vi "Emballage_BDD_chargement_IDArticle_GPAO_FLATPROP.vi"(0 "filenames":string[](array[string]), 1 "taille":i32, 2 "repertoireConfigs":path, 3 "Refnum Ch":refnum<vi>, 7 "entrée d'erreur (pas d'erreur)":errorcluster, 12 "progress":refnum<vi>) -> (10 "Code_Barre_Fixe":string, 14 "affiche_code_barre_client":string, 16 "codification":string, 17 "melange_des_lots_possible":string, 18 "Indice":string, 19 "id_article":string, 20 "clc_designation":string, 21 "affiche-no-client":string, 22 "Tableau en sortie":string[][](array[string]), 23 "Nb_valve_par_carton":string, 24 "tableau ajouté":string[](array[string]), 25 "suffixe":string, 26 "INDICE_REV":string, 27 "sortie d'erreur":errorcluster)   [LabVIEW 2020]
uses:
  Modules/FS/60_FS_Controles/60_FS_SetGet.ctl
panel:
  out "code_barre_fixe_fin":string
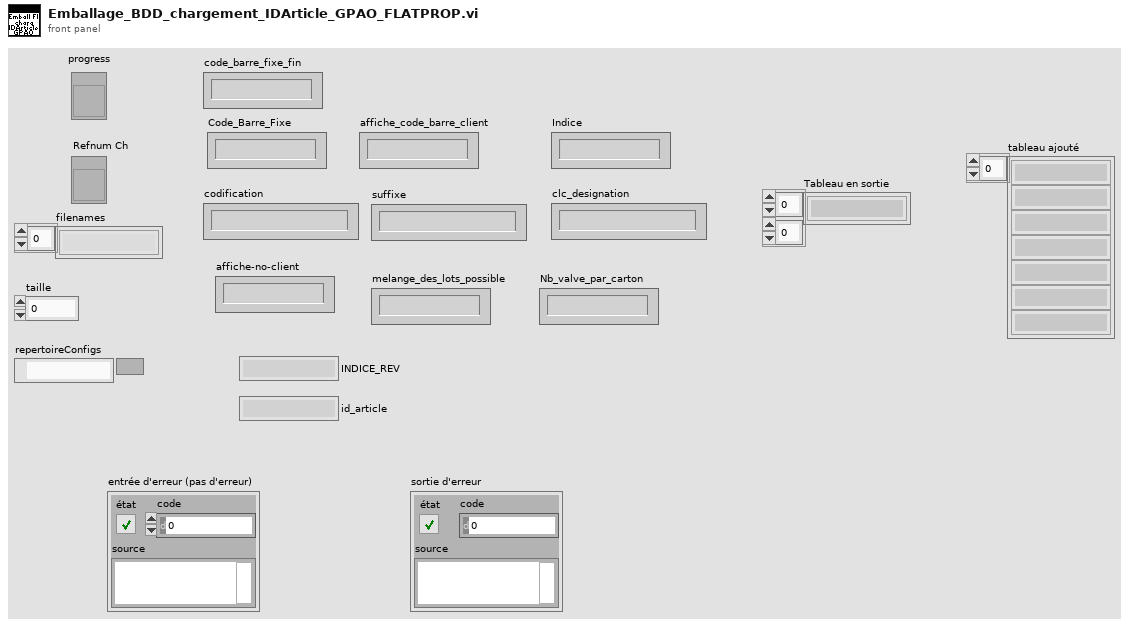
[diagram p1: front panel]
types:
  T1 = typedef "60_FS_SetGet.ctl" = enum16{"set", "get"}
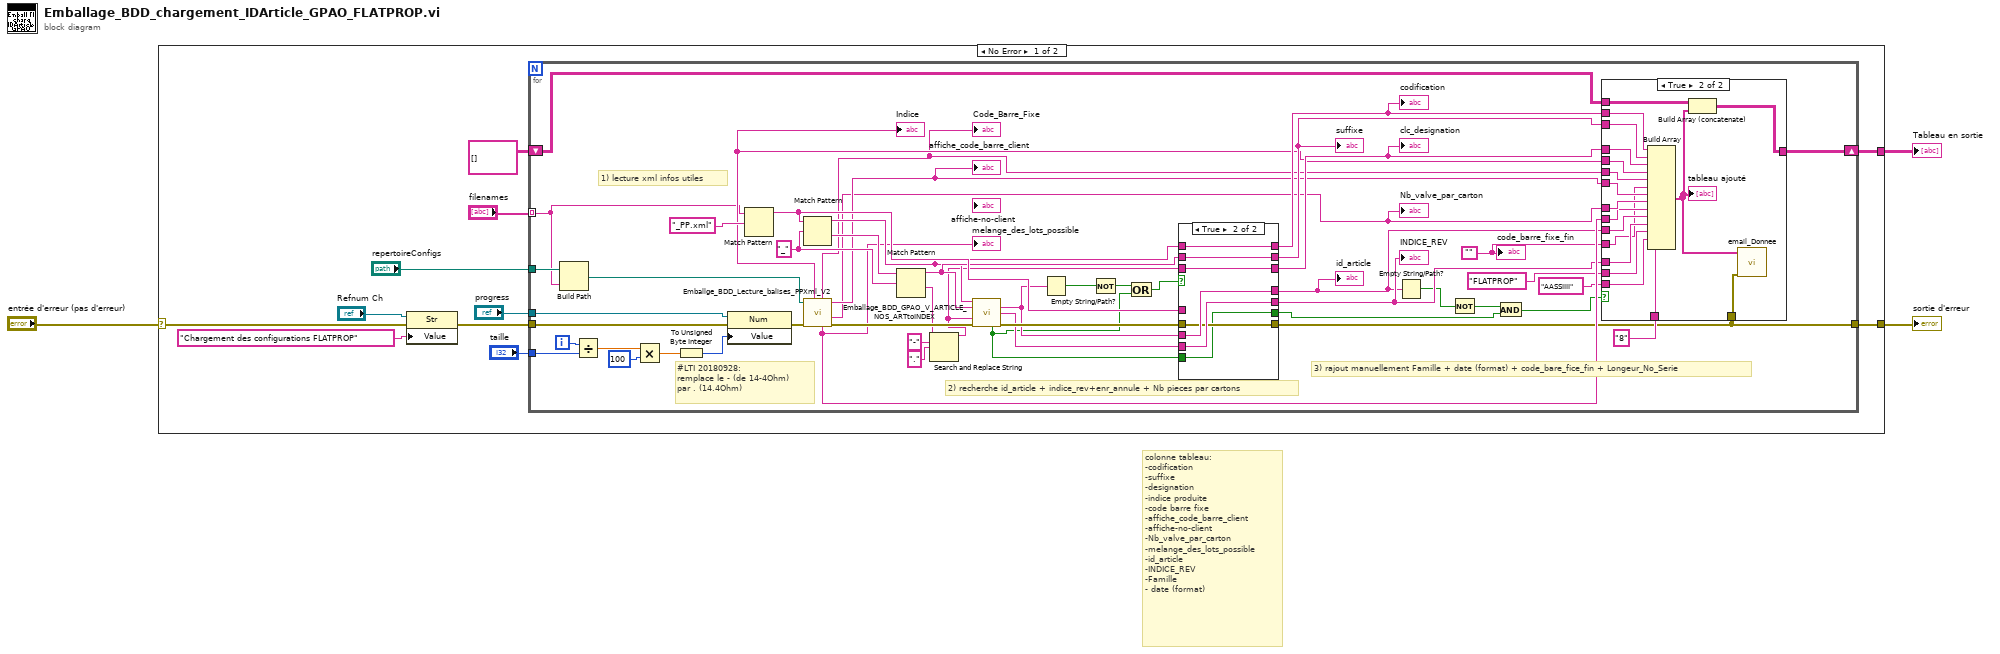
[diagram p0: block diagram]
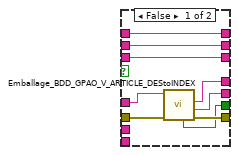
[diagram p3: hidden frame]
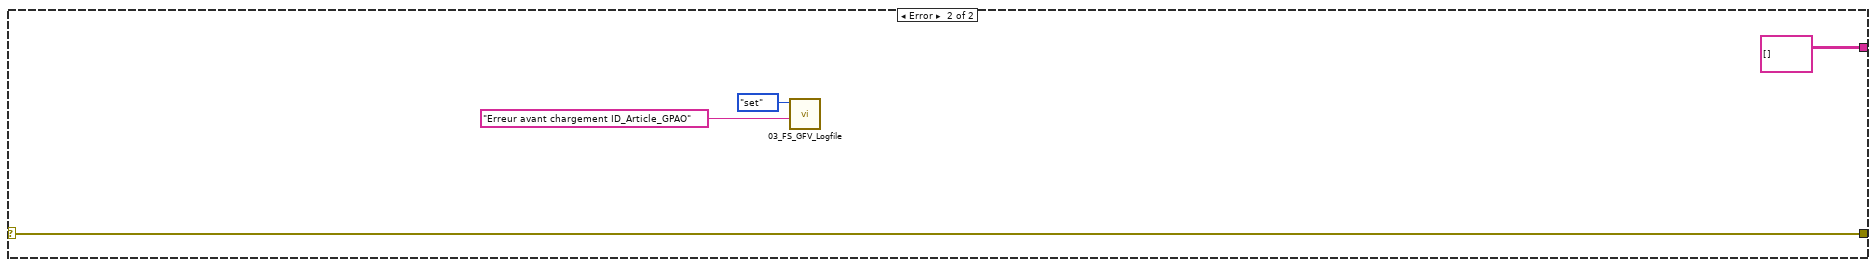
[diagram p4: hidden frame]
diagram:
  # "colonne tableau:\n-codification\n-suffixe\n-designation\n-indice produite\n-code barre fixe\n-affiche_code_barre_client\n-affiche-no-client\n-Nb_valve_par_carton\n-melange_des_lots_possible\n-id_article\n-INDICE_REV\n-Famille\n- date (format)"
  n1 = case shown="No Error" "entrée d'erreur (pas d'erreur)" {
    selector: "entrée d'erreur (pas d'erreur)" -> [w6 w104]
    tunnel: [w14 string[][] [] ("Tableau en entrée")] -> w3
    tunnel: [w9 w104] -> w1
    frame No Error {
      n2 = property class="Str"(reference="Refnum Ch", error in=w6, "Value"="Chargement des configurations FLATPROP" ("Valeur")) -> (error out=w5:errorcluster)  [unwired: 1 out]
      n3 = for {
        tunnel: "repertoireConfigs" -> [w65]
        tunnel: "filenames" -> [w19] mode=indexing
        tunnel: w5 -> [w35]
        tunnel: "taille" -> [w59]
        shift-right: [w38] -> w14
        shift-left: string[][] [] ("Tableau en entrée") -> [w39]
        tunnel: [w15] -> w9
        tunnel: "progress" -> [w33]
        i -> [w60]
        w23 = ""
        w51 = "_" ("expression régulière")
        # "#LTI 20180928:\nremplace le - (de 14-4Ohm)\npar . (14.4Ohm)"
        # "3) rajout manuellement Famille + date (format) + code_bare_fice_fin + Longeur_No_Serie"
        # "2) recherche id_article + indice_rev+enr_annule + Nb pieces par cartons"
        # "1) lecture xml infos utiles"
        n4 = Build Path(base path=w65, name or relative path=w19) -> (appended path=w64:path)
        n5 = Divide(x=w60, y=w59) -> (x/y=w61:dbl)
        n6 = Multiply(x=w61, y=u8 100) -> (x*y=w63:dbl)
        n7 = To Unsigned Byte Integer(number=w63) -> (unsigned 8bit integer=w36:u8)
        n8 = property class="Num"(reference=w33, error in=w35, "Value"=w36) -> (error out=w34:errorcluster)  [unwired: 1 out]
        n9 = Match Pattern(string=w19, regular expression="_PP.xml" ("expression régulière")) -> (before substring=w57:string)  [unwired: 1 in, 3 out]
        n10 = Match Pattern(string=w57, regular expression=w51) -> (before substring=w53:string, after substring=w52:string)  [unwired: 1 in, 2 out]
        n11 = call "Emballge_BDD_Lecture_balises_PPXml_V2.vi"("entrée d'erreur (pas d'erreur)"=w34, "appended path"=w64) -> ("sortie d'erreur"=w48:errorcluster, "Nb_valve_par_carton"=w16:string, "affiche_code_barre_client"=w42:string, "melange_des_lots_possible"=w41:string, "Code_Barre_Fixe"=w43:string, "Indice"=w44:string)  [unwired: 4 in]
        "affiche_code_barre_client" <- w42
        "melange_des_lots_possible" <- w41
        "Nb_valve_par_carton" <- w16
        "Code_Barre_Fixe" <- w43
        "Indice" <- w44
        n12 = Match Pattern(string=w52, regular expression=w51) -> (before substring=w54:string, after substring=w18:string)  [unwired: 1 in, 2 out]
        n13 = Search and Replace String(input string=w18, search string="-" ("chaîne recherchée"), replace string="." ("chaîne de remplacement (\"\")")) -> (result string=w17:string)  [unwired: 5 in, 3 out]
        n14 = call "Emballage_BDD_GPAO_V_ARTICLE_NOS_ARTtoINDEX.vi"("codification"=w53, "suffixe"=w54, "clc_designation"=w17, "error in (no error)"=w48) -> ("id_article"=w55:string, "INDICE_REV"=w56:string, "pce_non_annule"=w29:bool, "error out"=w58:errorcluster)  [unwired: 4 in, 4 out]
        n15 = Empty String/Path?(string/path=w55) -> (empty?=w49:bool)
        n16 = Not(x=w49) -> (.not. x?=w30:bool)
        n17 = Or(x=w30, y=w29) -> (x .or. y?=w31:bool)
        n18 = case shown="True" w31 {
          tunnel: w53 -> [w86 w100]
          tunnel: [w86 w100] -> w47
          tunnel: w54 -> [w87 w99]
          tunnel: [w87 w99] -> w46
          tunnel: w17 -> [w88 w98]
          tunnel: [w88 w98] -> w45
          tunnel: w55 -> [_ w97]
          tunnel: [w90 w97] -> w26
          tunnel: w56 -> [_ w96]
          tunnel: [w89 w96] -> w40
          tunnel: w57 -> [w93 _]
          tunnel: w58 -> [w92 w95]
          tunnel: [w91 w95] -> w15
          tunnel: [w85 w94] -> w27
          tunnel: w29 -> [_ w94]
          frame False {
            n19 = call "Emballage_BDD_GPAO_V_ARTICLE_DEStoINDEX.vi"("error in (no error)"=w92, "designation"=w93) -> ("error out"=w91:errorcluster, "INDICE_REV"=w89:string, "id_article"=w90:string, "pce_non_annule"=w85:bool)  [unwired: 4 in, 2 out]
          }
          frame True {
          }
        }
        "codification" <- w47
        "suffixe" <- w46
        "clc_designation" <- w45
        "id_article" <- w26
        "INDICE_REV" <- w40
        n20 = Empty String/Path?(string/path=w26) -> (empty?=w25:bool)
        n21 = Not(x=w25) -> (.not. x?=w24:bool)
        n22 = And(x=w24, y=w27) -> (x .and. y?=w28:bool)
        n23 = case shown="True" w28 {
          tunnel: w47 -> [_ w84]
          tunnel: w46 -> [_ w83]
          tunnel: w45 -> [_ w82]
          tunnel: w44 -> [_ w81]
          tunnel: w43 -> [_ w80]
          tunnel: w42 -> [_ w79]
          tunnel: w16 -> [_ w78]
          tunnel: w41 -> [_ w77]
          tunnel: w26 -> [_ w76]
          tunnel: w40 -> [_ w75]
          tunnel: w39 -> [w66 w74]
          tunnel: [w66 w73] -> w38
          tunnel: "FLATPROP" ("élément") -> [_ w72]
          tunnel: "AASSIIII" ("élément") -> [_ w71]
          tunnel: w23 -> [_ w70]
          tunnel: "8" ("élément") -> [_ w69]
          tunnel: w15 -> [_ w68]
          frame False {
            # "enregistrement annulé\npas afficher"
          }
          frame True {
            n24 = Build Array(w84, w83, w82, w81, w80, w70, w79, w78, w77, w76, w75, w72, w71, w69) -> (w67:string[])
            "tableau ajouté" <- w67
            n25 = Build Array (concatenate)(w74, w67) -> (w73:string[][])
            n26 = call "email_Donnee.vi"("entrée d'erreur (pas d'erreur)"=w68, "tableau_config"=w67) -> ()  [unwired: 9 in, 1 out]
          }
        }
        "code_barre_fixe_fin" <- w23
      }
    }
    frame Error {
      n27 = call "03_FS_GFV_Logfile.vi"("Chaîne"="Erreur avant chargement ID_Article_GPAO", "States"=60_FS_SetGet."set") -> ()  [unwired: 8 in, 2 out]
    }
  }
  "Tableau en sortie" <- w3
  "sortie d'erreur" <- w1
